vi "Add Combo Box Items.vi"(8 "error in (no error)":errorcluster, 10 "String Array":string[](array[string]), 11 "Items Refnum in":refnum<k24>) -> (0 "error out":errorcluster, 3 "Items Refnum Out":refnum<k24>)   [LabVIEW 2013, in "DataGrid.lvlib" / "DataGridView.lvclass"]
uses:
  DataGridView.lvclass
  System.Windows.Forms
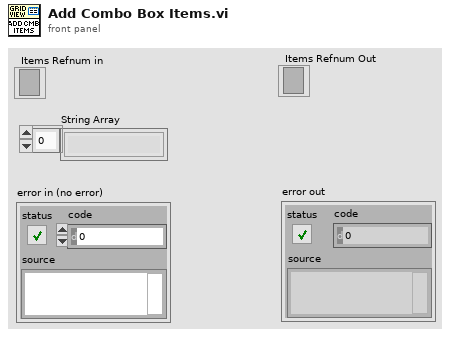
[diagram p1: front panel]
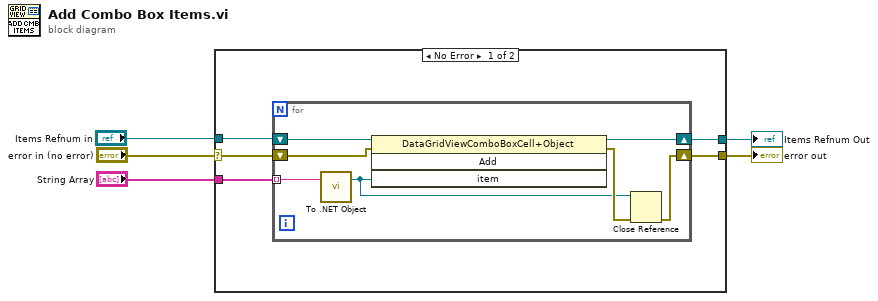
[diagram p0: block diagram]
diagram:
  n1 = case shown="No Error" "error in (no error)" {
    selector: "error in (no error)" -> [w6 w19]
    tunnel: "Items Refnum in" -> [w10 w18]
    tunnel: "String Array" -> [w9 _]
    tunnel: [w8 w19] -> w3
    tunnel: [w7 w18] -> w2
    frame No Error {
      n2 = for {
        tunnel: w9 -> [w16] mode=indexing
        shift-right: [w15] -> w7
        shift-left: w10 -> [w17]
        shift-right: [w12] -> w8
        shift-left: w6 -> [w13]
        n3 = call <vilib>:"To .NET Object.vi"("anything"=w16) -> (".NET object"=w11:refnum<k24>)  [unwired: 1 in, 1 out]
        n4 = invoke class="DataGridViewComboBoxCell+Object" method="Add"(reference=w17, error in=w13, "item"=w11) -> (reference out=w15:refnum<k24>, error out=w14:errorcluster)  [unwired: 1 in, 2 out]
        n5 = Close Reference(reference=w11, error in (no error)=w14) -> (error out=w12:errorcluster)
      }
    }
    frame Error {
    }
  }
  "error out" <- w3
  "Items Refnum Out" <- w2
